vi "Login-Window-Core.vi"(5 "Cluster":T1, 7 "PwdMgr":refnum<class "PwdMgr.lvclass">, 8 "Error in":errorcluster caption="Error in (no error)", 9 "Fit to Large Dec?(T)":bool=TRUE, 11 "Options":T2={"HideMain(T)"=TRUE, "RetryAllowed(T)"=TRUE, "LastUserToINI(T)"=TRUE, "Titlebar(T)"=TRUE}) -> (0 "Error out":errorcluster={"status"=TRUE, "code"=43, "source"="Operation cancelled by user."}, 1 "Valid User":bool, 3 "User Info":T3={"UserName"="", "Password"="", "Role"=enum."Admin"})   [LabVIEW 2020, in "Login-UI.lvlib"]
uses:
  Login-UI.lvlib
  _Typedef/User-Info.ctl
  _Typedef/User-Role.ctl
  Login-Options.ctl
  PwdMgr/PwdMgr.lvclass
  <vilib>/event_ctls.llb/eventvkey.ctl
  82dbac5f-f66d-497b-81a9-0f95a8baf484.vi
  <resource>/dialog/lvconfig.llb/LV Config Write String.vi
  <resource>/dialog/lvconfig.llb/LV Config Read String.vi
  <userlib>/NEVSTOP-Programming-Palette/_openG/_reuse_openG_nevstop.lvlib
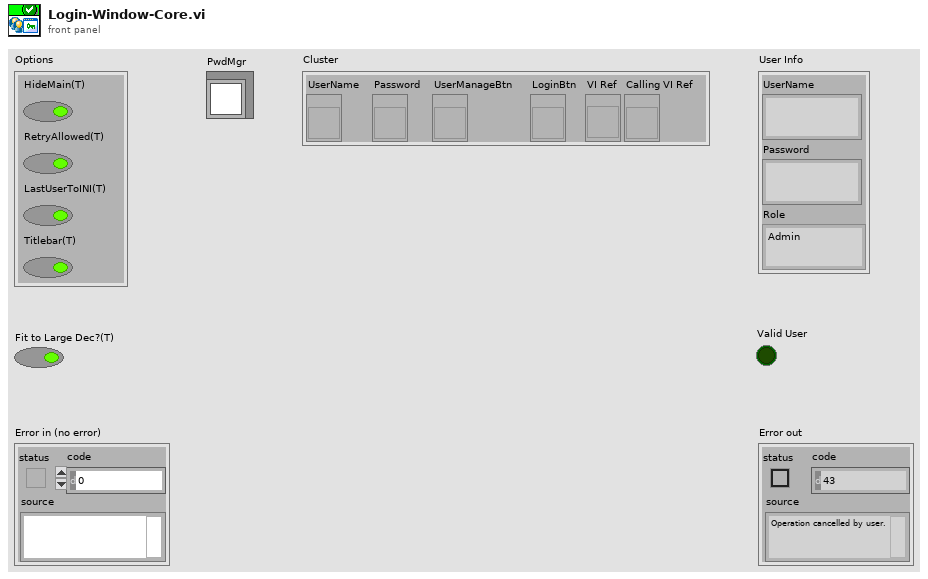
[diagram p1: front panel]
types:
  T1 = cluster{"UserName":refnum<vi>, "Password":refnum<vi>, "UserManageBtn":refnum<vi>, "LoginBtn":refnum<vi>, "VI Ref":refnum<vi>, "Calling VI Ref":refnum<vi>}
  T2 = typedef "Login-UI.lvlib/Login-Options.ctl" = cluster{"HideMain(T)":bool, "RetryAllowed(T)":bool, "LastUserToINI(T)":bool, "Titlebar(T)":bool}
  T3 = typedef "Login-UI.lvlib/User-Info.ctl" = cluster{"UserName":string, "Password":string, "Role":T4}
  T4 = typedef "Login-UI.lvlib/User-Role.ctl" = enum16{"INVALID", "Operator", "Engineer", "Admin", "Anonymous"}
  T5 = typedef "eventvkey.ctl" = enum16{"ASCII", "Enter", "Return", "Shift", "Ctrl", "Alt", "Cmd", "Opt", "Caps", "NumLock", "Clear", "Break", "Up", "Down", "Left", "Right", "Insert", "Delete", "Home", "End", "PageUp", "PageDown", "Escape", "Help", "Pause", "ScrollLock", "F1", "F2", "F3", "F4", "F5", "F6", "F7", "F8", "F9", "F10", "F11", "F12", "F13", "F14", "F15", "F16", "F17", "F18", "F19", "F20", "F21", "F22", "F23", "F24", "Play", "VolumeUp", "VolumeDown", "Mute", "Two Byte Char"}
  T6 = enum32{"Invalid", "Standard", "Closed", "Hidden", "Minimized", "Maximized"}
  T7 = enum32{"invalid app kind", "Development System", "Run Time System", "Student Edition", "Embedded LabVIEW", "Evaluation", "Custom"}
  T8 = cluster{"Core":cluster{"Current VI Reference":refnum<vi>, "Close Panel on Exit?":bool}, "Options":T2, "Calling VI's Ref":refnum<vi>, "Calling VI's FP.State":enum32{"Invalid", "Standard", "Closed", "Hidden", "Minimized", "Maximized"}, "Result":cluster{"LoginSuccess":bool, "error":errorcluster, "User Info":T3}, "UserName":string, "Password":string, "StringRefs":refnum<vi>[]}
  T9 = cluster{"LoginSuccess":bool, "error":errorcluster, "User Info":T3}
  T10 = cluster{"Current VI Reference":refnum<vi>, "Close Panel on Exit?":bool}
  T11 = cluster{bool, "code":i32, "String to Prepend to source (\"\")":string}
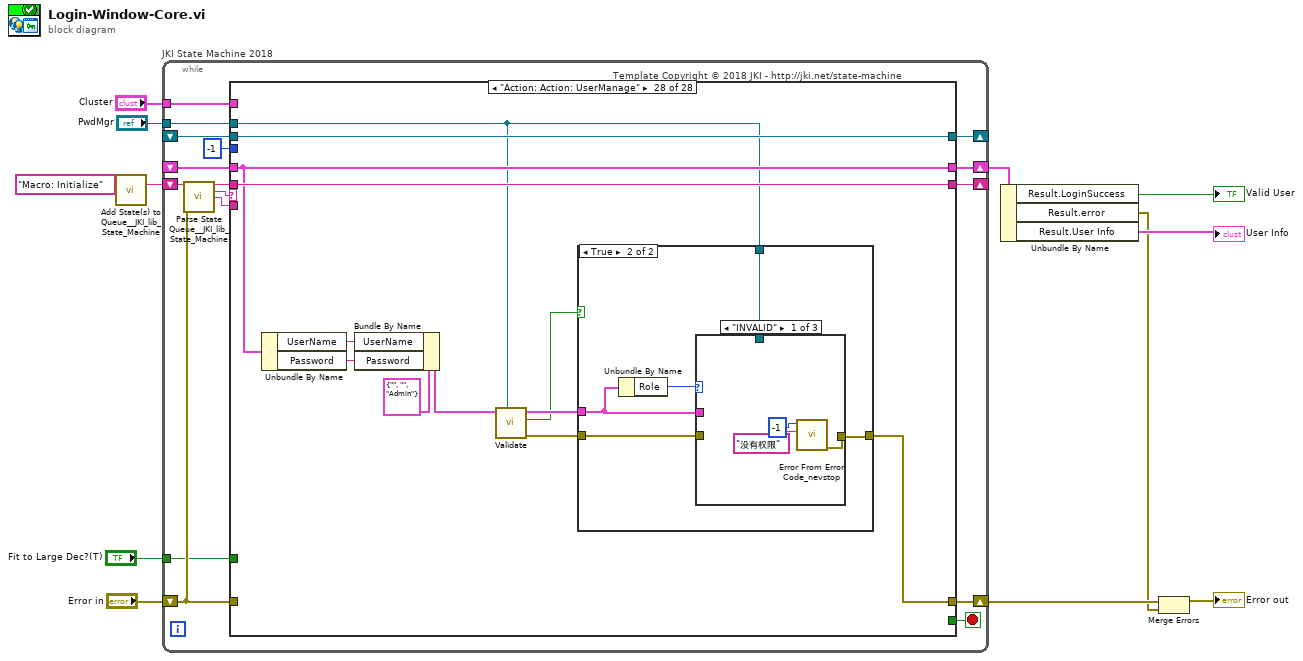
[diagram p0: block diagram]
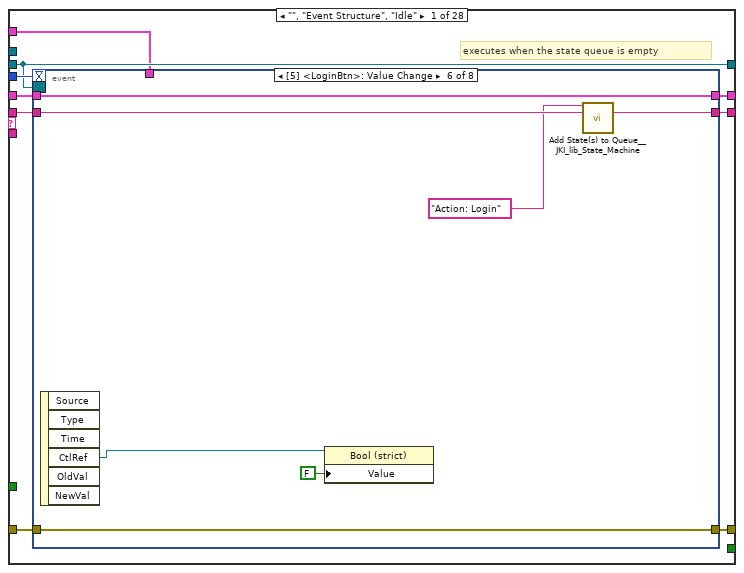
[diagram p2: hidden frame]
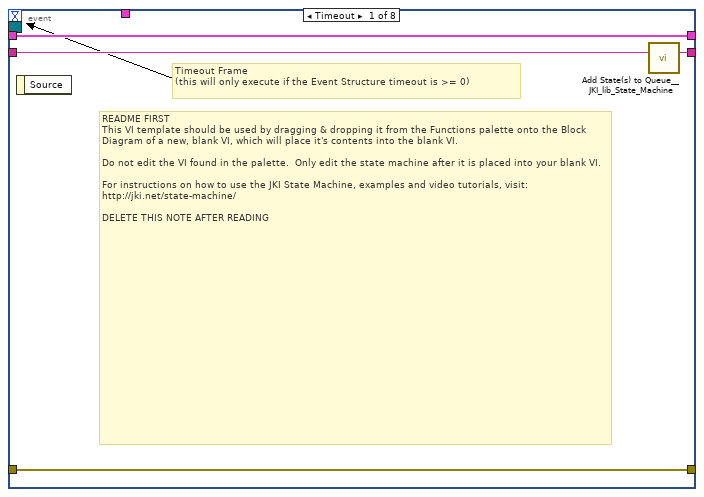
[diagram p3: hidden frame]
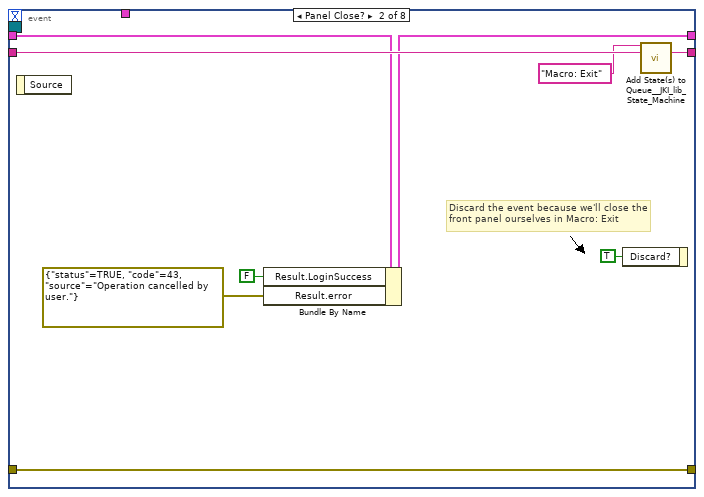
[diagram p4: hidden frame]
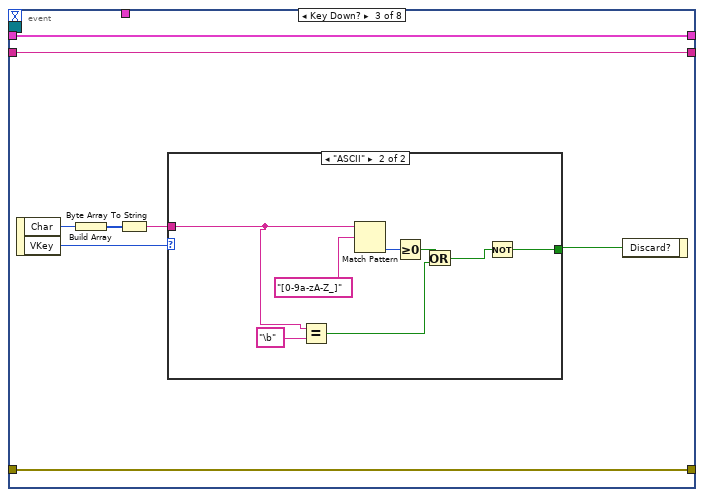
[diagram p5: hidden frame]
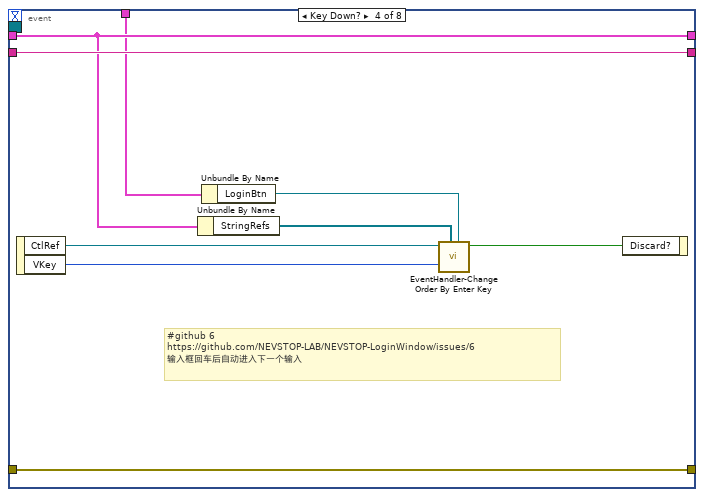
[diagram p7: hidden frame]
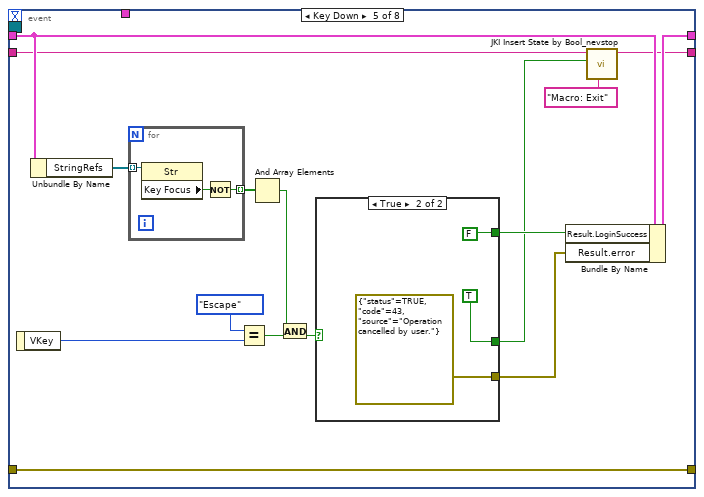
[diagram p8: hidden frame]
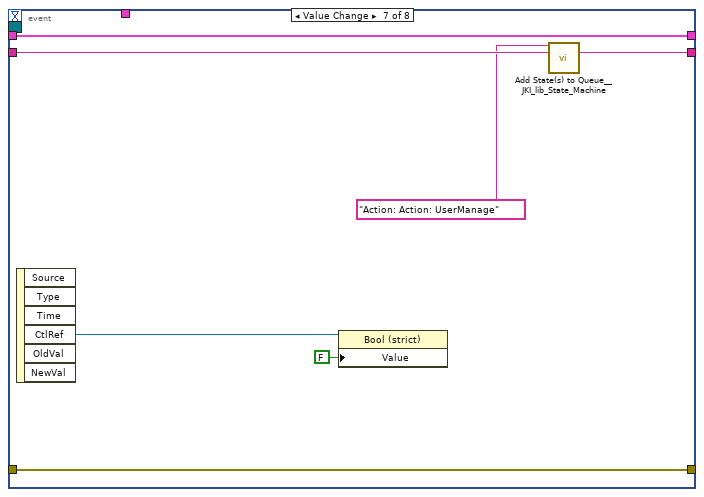
[diagram p10: hidden frame]
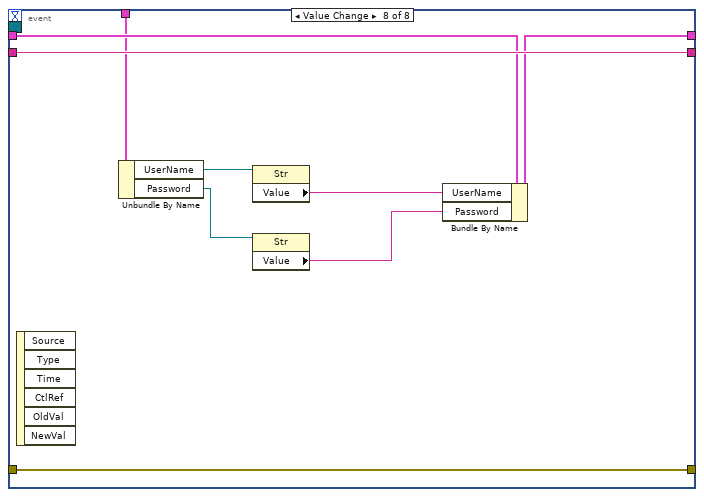
[diagram p11: hidden frame]
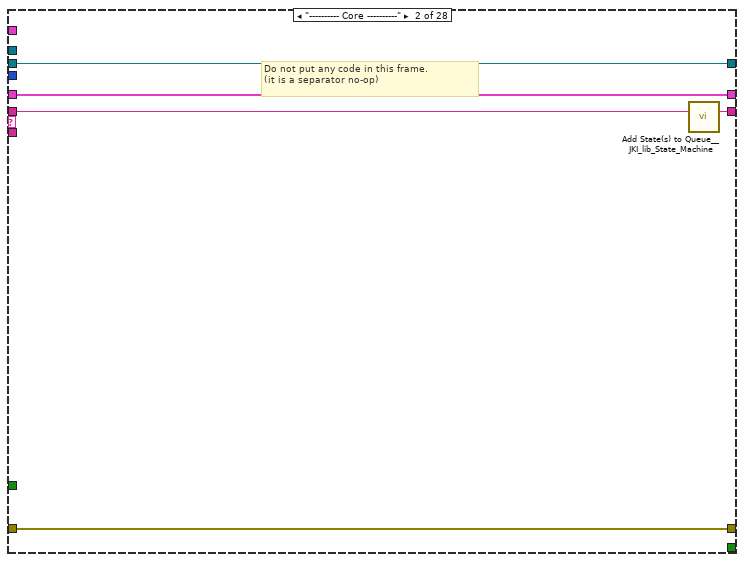
[diagram p12: hidden frame]
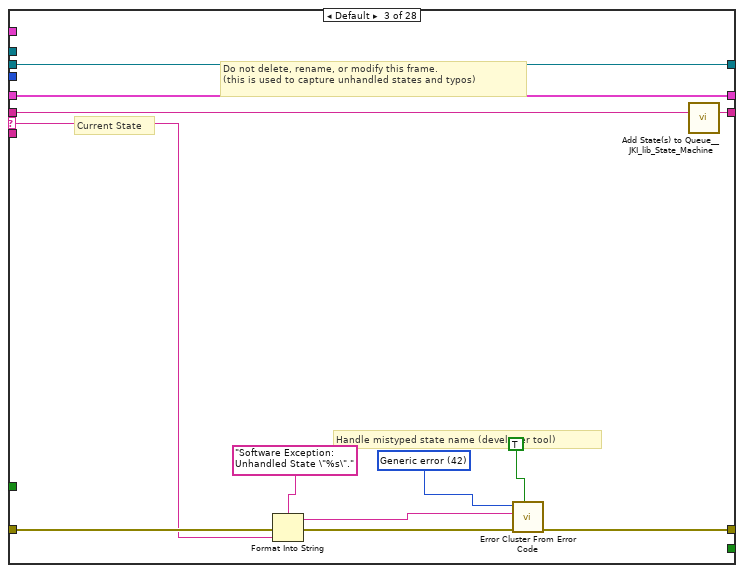
[diagram p13: hidden frame]
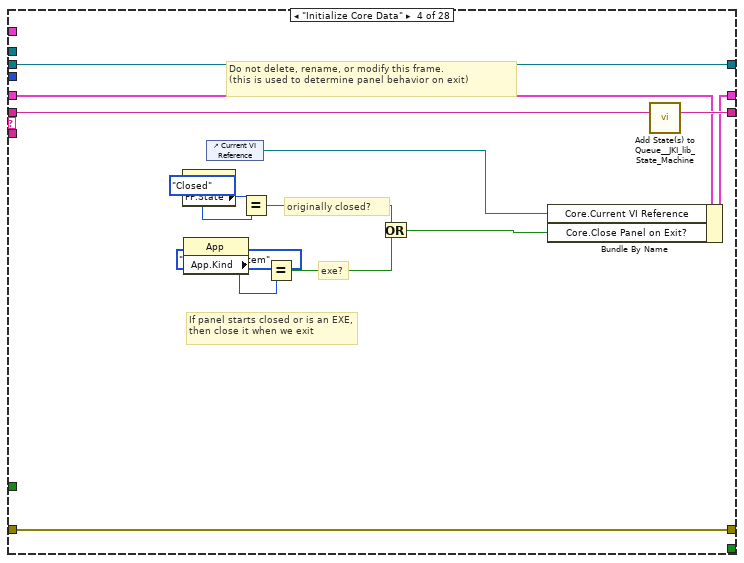
[diagram p14: hidden frame]
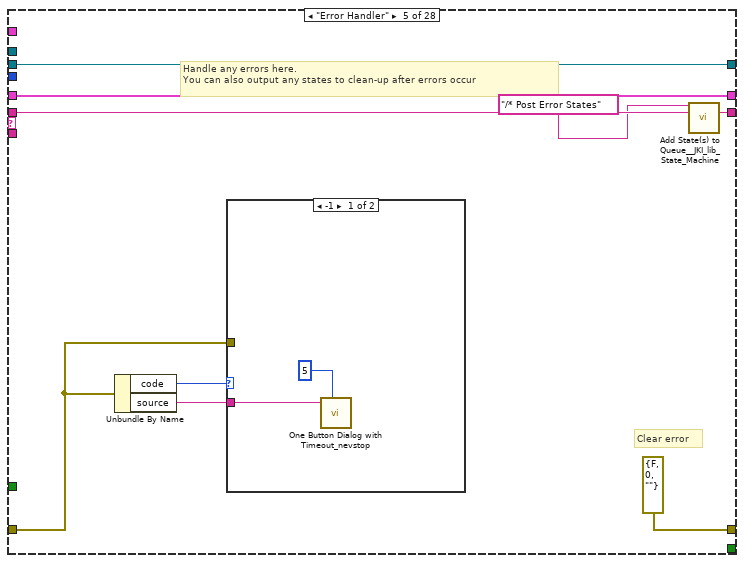
[diagram p15: hidden frame]
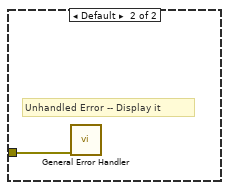
[diagram p16: hidden frame]
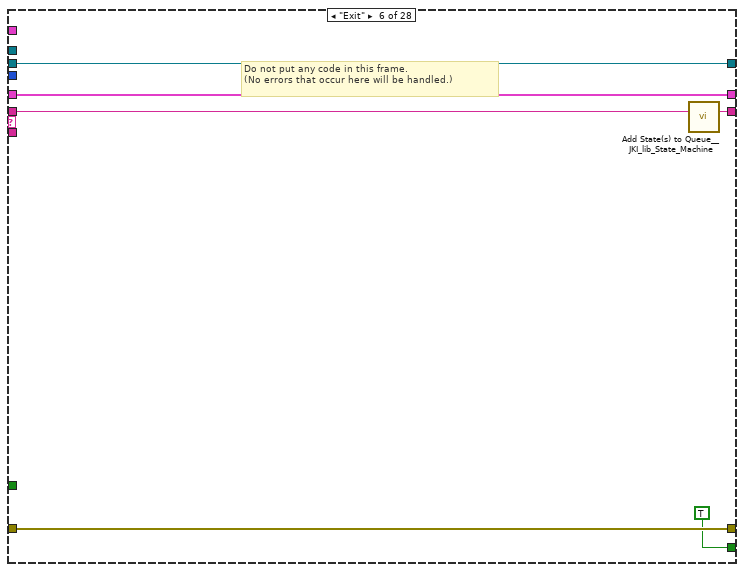
[diagram p17: hidden frame]
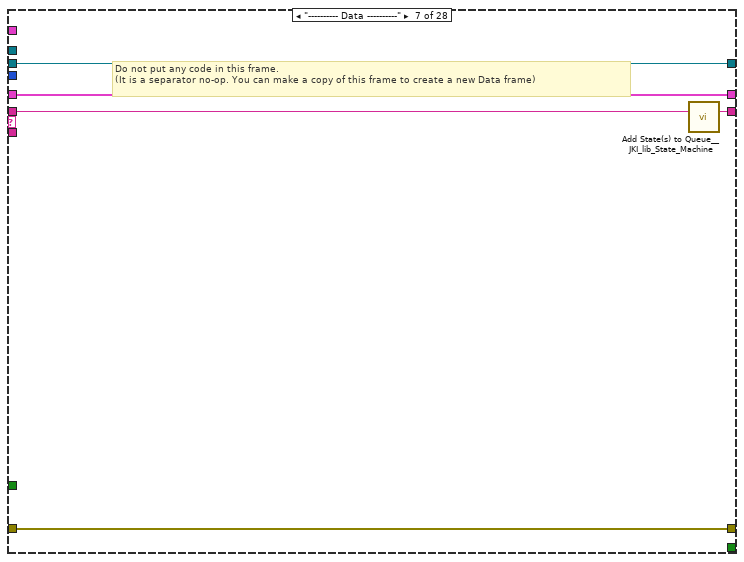
[diagram p18: hidden frame]
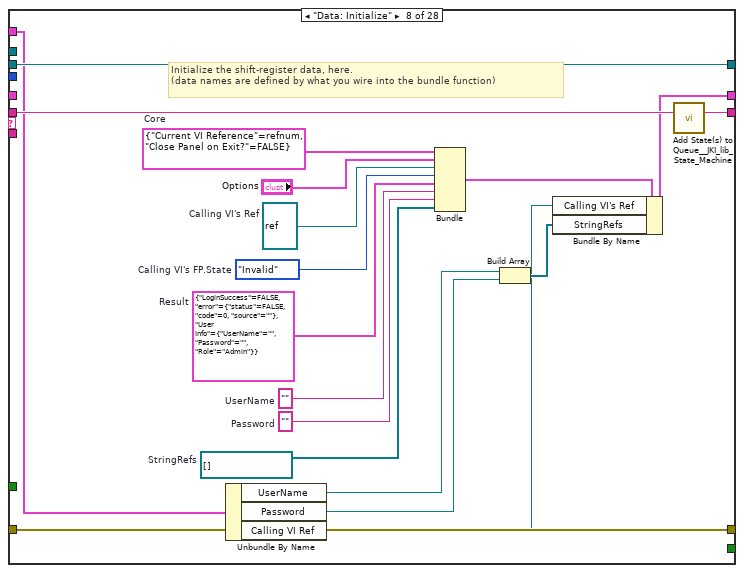
[diagram p19: hidden frame]
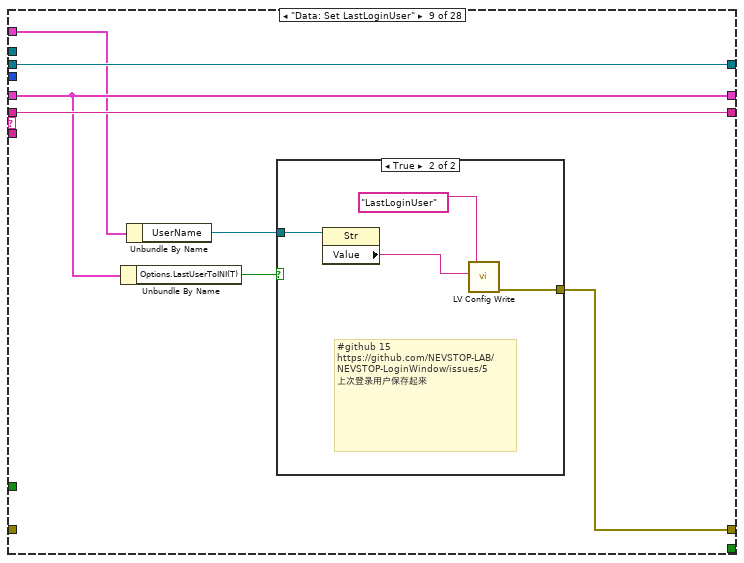
[diagram p20: hidden frame]
diagram:
  n1 = call <vilib>:"Add State(s) to Queue__JKI_lib_State_Machine.vi"("State(s) in (\"\")"="Macro: Initialize") -> ("States Out"=w10:string)  [unwired: 14 in]
  n2 = while "JKI State Machine 2018" {
    shift-right: [w21] -> w7
    shift-left: _ -> [w20]
    shift-right: [w24] -> w8
    shift-left: "Error in" -> [w18]
    shift-right: [w23] -> _
    shift-left: w10 -> [w25]
    shift-right: [w17] -> _
    shift-left: _ -> [w16]
    tunnel: "PwdMgr" -> [w15]
    tunnel: "Cluster" -> [w14]
    tunnel: "Fit to Large Dec?(T)" -> [w13]
    stop <- w22 stop-if-true
    # "Template Copyright © 2018 JKI - http://jki.net/state-machine"
    n3 = call <vilib>:"Parse State Queue__JKI_lib_State_Machine.vi"("State Queue"=w25, "Error In (no error)"=w18) -> ("Remaining States"=w27:string, "Current State"=w28:string, "Arguments"=w26:string)  [unwired: 11 in]
    n4 = case shown="\"Action: Action: UserManage\"" w28 {
      selector: w28 -> [_ _ w127 _ _ _ _ _ _ _ _ _ _ _ _ _ _ _ _ _ _ _ _ _ _ _ _ _]
      tunnel: w27 -> [w37 w125 w131 w151 w160 w169 w174 w193 w200 w211 w216 w230 w236 w241 w251 w261 w273 w347 w359 w373 w386 w392 w398 w409 w414 w433 w447 w459]
      tunnel: w26 -> [_ _ _ _ _ _ _ _ _ _ _ _ _ _ _ w256 w267 _ _ _ _ _ _ _ _ _ _ _]
      tunnel: w20 -> [w35 w122 w129 w144 w157 w167 w171 _ w198 w206 w213 w219 w234 w238 w249 w259 w269 w345 w356 w371 w384 w389 w395 w406 w411 w425 w443 w456]
      tunnel: [w34 w123 w133 w148 errorcluster {"status"=FALSE, "code"=0, "source"=""} ("error out") w166 w172 w190 w196 w207 w214 w227 w231 w239 w246 w257 w270 w343 w360 w374 w387 w390 w396 w407 w412 w431 w445 w452] -> w24
      tunnel: w18 -> [w33 w123 w132 w148 w154 w166 w172 w190 _ w208 w214 _ w232 w239 _ w258 w271 _ w360 w374 w387 w390 w396 w407 w412 w431 w445 _]
      tunnel: [w36 w124 w130 w150 w159 w168 w173 w192 w200 w210 w215 w229 w235 w240 w250 w260 w272 w347 w359 w373 w386 w391 w397 w408 w413 w432 w446 w459] -> w23
      tunnel: [_ _ _ _ _ TRUE _ _ _ _ _ _ _ _ _ _ _ _ _ _ _ _ _ _ _ _ _ _] -> w22
      tunnel: [w32 w122 w129 w149 w157 w167 w171 w184 w198 w206 w213 w219 w234 w238 w249 w259 w269 w345 w354 w371 w384 w389 w395 w406 w411 w421 w441 w456] -> w21
      tunnel: -1 ("Timeout") -> [w31 _ _ _ _ _ _ _ _ _ _ _ _ _ _ _ _ _ _ _ _ _ _ _ _ _ _ _]
      tunnel: [w30 w121 w126 w138 w155 w164 w170 w188 w199 w205 w212 w228 w233 w237 w248 w255 w266 w346 w358 w372 w385 w388 w393 w399 w410 w430 w444 w458] -> w17
      tunnel: w16 -> [w30 w121 w126 w138 w155 w164 w170 w188 w199 w205 w212 _ w233 w237 w248 w255 w266 w346 w358 w372 w385 w388 w393 w399 w410 w430 w444 w458]
      tunnel: w15 -> [_ _ _ _ _ _ _ _ _ _ _ _ _ _ _ _ _ _ _ _ _ _ _ _ _ w418 _ w448]
      tunnel: w14 -> [w29 _ _ _ _ _ _ w178 w195 _ _ w226 _ _ w244 _ _ w342 _ _ _ _ _ _ _ _ _ _]
      tunnel: w13 -> [_ _ _ _ _ _ _ _ _ _ _ _ _ _ w242 _ _ _ _ _ _ _ _ _ _ _ _ _]
      frame "", "Event Structure", "Idle" {
        # "executes when the state queue is empty"
        n5 = event shown="[5] <LoginBtn>: Value Change" {
          selector: w30 -> [_ _ _ _ _ _ _ _]
          dyn-events: _ -> [_ _ _ _ _ _ _ _]
          timeout: w31 -> [_ _ _ _ _ _ _ _]
          tunnel: w37 -> [w41 w50 w58 w75 w78 w101 w108 w120]
          tunnel: [w40 w49 w58 w75 w79 w102 w109 w120] -> w36
          tunnel: w35 -> [w38 w47 w56 w70 w84 w103 w110 w118]
          tunnel: [w39 w48 w57 w74 w91 w104 w111 w119] -> w34
          tunnel: w33 -> [w39 w48 w57 w74 w91 w104 w111 w119]
          tunnel: [w38 w44 w56 w70 w82 w103 w110 w117] -> w32
          tunnel: w29 -> [_ _ _ w68 _ _ _ w116]
          event Timeout {
            # "README FIRST\nThis VI template should be used by dragging & dropping it from the Functions palette onto the Block Diagram of a new, blank VI, which will place it's contents into the blank VI.\n\nDo not edit the VI found in the palette.  Only edit the state machine after it is placed into your blank VI.\n\nFor instructions on how to use the JKI State Machine, examples and video tutorials, visit:\nhttp://jki.net/state-machine/\n\nDELETE THIS NOTE AFTER READING"
            # "Timeout Frame\n(this will only execute if the Event Structure timeout is >= 0)"
            n6 = event-data() -> ()  [unwired: 1 in, 1 out]
            n7 = call <vilib>:"Add State(s) to Queue__JKI_lib_State_Machine.vi"("State(s) in (\"\")"=w41) -> ("States Out"=w40:string)  [unwired: 14 in]
          }
          event Panel Close? {
            # "Discard the event because we'll close the front panel ourselves in Macro: Exit"
            n8 = event-data() -> ()  [unwired: 1 in, 1 out]
            n9 = Bundle By Name(cluster=w47, "Result.LoginSuccess"=FALSE, "Result.error"=errorcluster {"status"=TRUE, "code"=43, "source"="Operation cancelled by user."} ("error in")) -> (w44:T8)
            n10 = event-data("Discard?"=TRUE) -> ()  [unwired: 1 in, 1 out]
            n11 = call <vilib>:"Add State(s) to Queue__JKI_lib_State_Machine.vi"("State(s) in Front (\"\")"="Macro: Exit", "State(s) in (\"\")"=w50) -> ("States Out"=w49:string)  [unwired: 13 in]
          }
          event Key Down? {
            n12 = event-data() -> ("Char"=w53:i16, "VKey"=w52:T5)  [unwired: 1 in]
            n13 = Build Array(w53) -> (w54:i16[])
            n14 = Byte Array To String(unsigned byte array=w54) -> (string=w55:string)
            n15 = case shown="\"ASCII\"" w52 {
              tunnel: [_ w59] -> w51
              tunnel: w55 -> [_ w62]
              frame Default {
              }
              frame "ASCII" {
                n16 = Equal?(x=w62, y="\b" ("regular expression")) -> (x = y?=w60:bool)
                n17 = Match Pattern(string=w62, regular expression="[0-9a-zA-Z_]") -> (offset past match=w65:i32)  [unwired: 1 in, 3 out]
                n18 = Greater Or Equal To 0?(x=w65) -> (x >= 0?=w64:bool)
                n19 = Or(x=w64, y=w60) -> (x .or. y?=w61:bool)
                n20 = Not(x=w61) -> (.not. x?=w59:bool)
              }
            }
            n21 = event-data("Discard?"=w51) -> ()  [unwired: 1 in, 1 out]
          }
          event Key Down? {
            # "#github 6\nhttps://github.com/NEVSTOP-LAB/NEVSTOP-LoginWindow/issues/6\n输入框回车后自动进入下一个输入"
            n22 = event-data() -> ("CtlRef"=w72:refnum<vi>, "VKey"=w73:T5)  [unwired: 1 in]
            n23 = Unbundle By Name(w70) -> ("StringRefs"=w69:refnum<vi>[])
            n24 = Unbundle By Name(w68) -> ("LoginBtn"=w67:refnum<vi>)
            n25 = call "EventHandler-Change Order By Enter Key.vi"("Next Ctrl"=w67, "Controls for changing order"=w69, "VKey"=w73, "Event Control"=w72) -> ("Discard?"=w71:bool)  [unwired: 7 in]
            n26 = event-data("Discard?"=w71) -> ()  [unwired: 1 in, 1 out]
          }
          event Key Down {
            n27 = event-data() -> ("VKey"=w85:T5)  [unwired: 1 in]
            n28 = Unbundle By Name(w84) -> ("StringRefs"=w83:refnum<vi>[])
            n29 = for {
              tunnel: w83 -> [w94] mode=indexing
              tunnel: [w92] -> w89 mode=indexing
              n30 = property class="Str"(reference=w94) -> ("Key Focus"=w93:bool)  [unwired: 1 in, 2 out]
              n31 = Not(x=w93) -> (.not. x?=w92:bool)
            }
            n32 = Equal?(x=eventvkey."Escape", y=w85) -> (x = y?=w87:bool)
            n33 = And Array Elements(Boolean array=w89) -> (logical AND=w90:bool)
            n34 = And(x=w90, y=w87) -> (x .and. y?=w88:bool)
            n35 = case shown="True" w88 {
              tunnel: [_ TRUE ("Discard?")] -> w77
              tunnel: [_ FALSE ("Discard?")] -> w81
              tunnel: [_ errorcluster {"status"=TRUE, "code"=43, "source"="Operation cancelled by user."} ("error in")] -> w80
              frame False {
              }
              frame True {
              }
            }
            n36 = Bundle By Name(cluster=w84, "Result.LoginSuccess"=w81, "Result.error"=w80) -> (w82:T8)
            n37 = call <userlib>:"JKI Insert State by Bool_nevstop.vi"("TRUE(Empty)"="Macro: Exit", "Bool"=w77, "Remaining States"=w78) -> ("States Out"=w79:string)  [unwired: 8 in]
          }
          event Value Change {
            n38 = event-data() -> ("CtlRef"=w99:refnum<vi>)  [unwired: 1 in, 5 out]
            n39 = property class="Bool (strict)"(reference=w99, "Value"=FALSE) -> ()  [unwired: 1 in, 2 out]
            n40 = call <vilib>:"Add State(s) to Queue__JKI_lib_State_Machine.vi"("State(s) in Front (\"\")"="Action: Login" ("State(s) in Front (\"\")"), "State(s) in (\"\")"=w101) -> ("States Out"=w102:string)  [unwired: 13 in]
          }
          event Value Change {
            n41 = event-data() -> ("CtlRef"=w106:refnum<vi>)  [unwired: 1 in, 5 out]
            n42 = property class="Bool (strict)"(reference=w106, "Value"=FALSE) -> ()  [unwired: 1 in, 2 out]
            n43 = call <vilib>:"Add State(s) to Queue__JKI_lib_State_Machine.vi"("State(s) in Front (\"\")"="Action: Action: UserManage" ("State(s) in Front (\"\")"), "State(s) in (\"\")"=w108) -> ("States Out"=w109:string)  [unwired: 13 in]
          }
          event Value Change {
            n44 = event-data() -> ()  [unwired: 1 in, 6 out]
            n45 = Unbundle By Name(w116) -> ("UserName"=w115:refnum<vi>, "Password"=w114:refnum<vi>)
            n46 = property class="Str"(reference=w115) -> ("Value"=w112:string)  [unwired: 1 in, 2 out]
            n47 = property class="Str"(reference=w114) -> ("Value"=w113:string)  [unwired: 1 in, 2 out]
            n48 = Bundle By Name(cluster=w118, "UserName"=w112, "Password"=w113) -> (w117:T8)
          }
        }
      }
      frame "---------- Core ----------" {
        # "Do not put any code in this frame.\n(it is a separator no-op)"
        n49 = call <vilib>:"Add State(s) to Queue__JKI_lib_State_Machine.vi"("State(s) in (\"\")"=w125) -> ("States Out"=w124:string)  [unwired: 14 in]
      }
      frame Default {
        w136 = 42 items=["No error", "Argument error", "Memory is full", "Out of zone", "End of file", "File already open", "Generic file I/O error", "File not found", "File permission error", "Disk is full", "Duplicate path", "Too many files open", "System feature not enabled", "Resource file not found", "Cannot add resource", "Resource not found", "Image not found", "Image memory error", "Pen does not exist", "Config type invalid", "Config token not found", "Config parse error", "Config memory error", "Bad external code format", "Bad external code offset", "External code not present", "Null window", "Destroy window error", "Null menu", "Print aborted", "Bad print record", "Print driver error", "Windows error during printing", "Memory error during printing", "Print dialog error", "Generic print error", "Invalid device refnum", "Device not found", "Device parameter error", "Device unit error", "Cannot open device", "Device call aborted", "Generic error", "Cancelled by user", "Object ID too low", "Object ID too high", "Object not in heap", "Unknown heap", "Unknown object (invalid DefProc)", "Unknown object (DefProc not in table)", "Message out of range", "Invalid (null) method", "Unknown message", "Manager call not supported", "Bad address", "Network operation in progress", "Network operation timed out", "Connection is busy", "Network attribute not supported", "Network error", "Address in use", "System out of memory", "Connection aborted", "Connection refused", "Not connected", "Already connected", "Connection closed", "Initialization error (interapplication manager)", "Bad occurrence", "Wait on unbound occurrence handler", "Occurrence queue overflow", "Datalog type conflict", "Unused", "Unrecognized type (interapplication manager)", "Memory corrupt", "Failed to make temporary DLL", "Old CIN version", "Drag socket not found", "Failed to load drop-object", "Failed to register OLE object", "Failed to release OLE object", "Format specifier type mismatch", "Unknown format specifier", "Too few format specifiers", "Too many format specifiers", "Scan failed", "Newer CIN version", "Error converting to variant", "Runtime menu error", "Password tampered", "Variant attribute not found", "Incompatible variant data type", "Event data is not available", "Event Store is not present", "Occurrence is not found", "Event Queue is not created", "Event info is not available", "Refnum passed is NULL", "Error retrieving Class GUID", "Error retrieving CoClass GUID", "Error retrieving TypeLib GUID.", "Bad built application magic bytes.", "Specific driver is different from the specific driver associated with the Logical Name.", "There is no session opened to the class driver.", "Max Error", "MAX - Error with config objects", "MAX - Error loading configuration", "MAX - Group not supported"]
        # "Current State"
        # "Do not delete, rename, or modify this frame.\n(this is used to capture unhandled states and typos)"
        # "Handle mistyped state name (developer tool)"
        n50 = Format Into String(format string="Software Exception: Unhandled State \"%s\"." ("message"), error in=w132, w127) -> (resulting string=w135:string, error out=w134:errorcluster)  [unwired: 1 in]
        n51 = call <vilib>:"Error Cluster From Error Code.vi"("show call chain? (False)"=TRUE, "error in (no error)"=w134, "error message (\"\")"=w135, "error code (0)"=w136) -> ("error out"=w133:errorcluster)  [unwired: 5 in]
        n52 = call <vilib>:"Add State(s) to Queue__JKI_lib_State_Machine.vi"("State(s) in (\"\")"=w131) -> ("States Out"=w130:string)  [unwired: 14 in]
      }
      frame "Initialize Core Data" {
        # "Do not delete, rename, or modify this frame.\n(this is used to determine panel behavior on exit)"
        # "originally closed?"
        # "exe?"
        # "If panel starts closed or is an EXE, then close it when we exit"
        n53 = property class="VI"() -> ("FP.State"=w141:T6)  [unwired: 2 in, 2 out]
        n54 = property class="App"() -> ("App.Kind"=w147:T7)  [unwired: 2 in, 2 out]
        n55 = control-ref of="Current VI Reference"() -> (w142:refnum<vi>)
        n56 = Equal?(x=w141, y=T6."Closed" ("Front Panel Window:State")) -> (x = y?=w139:bool)
        n57 = Equal?(x=w147, y=T7."Run Time System" ("Application:Kind")) -> (x = y?=w145:bool)
        n58 = Or(x=w139, y=w145) -> (x .or. y?=w143:bool)
        n59 = Bundle By Name(cluster=w144, "Core.Current VI Reference"=w142, "Core.Close Panel on Exit?"=w143) -> (w149:T8)
        n60 = call <vilib>:"Add State(s) to Queue__JKI_lib_State_Machine.vi"("State(s) in (\"\")"=w151) -> ("States Out"=w150:string)  [unwired: 14 in]
      }
      frame "Error Handler" {
        # "Handle any errors here.\nYou can also output any states to clean-up after errors occur"
        # "Clear error"
        n61 = Unbundle By Name(w154) -> ("code"=w153:i32, "source"=w152:string)
        n62 = case shown="-1" w153 {
          tunnel: w154 -> [_ w163]
          tunnel: w152 -> [w162 _]
          frame -1 {
            n63 = call <userlib>:"One Button Dialog with Timeout_nevstop.vi"("message"=w162, "Btn Timeout(-1 s)"=5) -> ()  [unwired: 7 in, 1 out]
          }
          frame Default {
            # "Unhandled Error -- Display it"
            n64 = call <vilib>:"General Error Handler.vi"("error in (no error)"=w163) -> ()  [unwired: 10 in, 5 out]
          }
        }
        n65 = call <vilib>:"Add State(s) to Queue__JKI_lib_State_Machine.vi"("State(s) in Front (\"\")"="/* Post Error States", "State(s) in (\"\")"=w160) -> ("States Out"=w159:string)  [unwired: 13 in]
      }
      frame "Exit" {
        # "Do not put any code in this frame.\n(No errors that occur here will be handled.)"
        n66 = call <vilib>:"Add State(s) to Queue__JKI_lib_State_Machine.vi"("State(s) in (\"\")"=w169) -> ("States Out"=w168:string)  [unwired: 14 in]
      }
      frame "---------- Data ----------" {
        # "Do not put any code in this frame.\n(It is a separator no-op. You can make a copy of this frame to create a new Data frame)"
        n67 = call <vilib>:"Add State(s) to Queue__JKI_lib_State_Machine.vi"("State(s) in (\"\")"=w174) -> ("States Out"=w173:string)  [unwired: 14 in]
      }
      frame "Data: Initialize" {
        w180 = refnum<vi>[] []  # StringRefs
        w181 = ""  # Password
        w182 = ""  # UserName
        w183 = T9 {"LoginSuccess"=FALSE, "error"={"status"=FALSE, "code"=0, "source"=""}, "User Info"={"UserName"="", "Password"="", "Role"=enum."Admin"}}  # Result
        w185 = T6."Invalid"  # Calling VI's FP.State
        w186 = refnum<vi> refnum  # Calling VI's Ref
        w189 = T10 {"Current VI Reference"=refnum, "Close Panel on Exit?"=FALSE}  # Core
        # "Initialize the shift-register data, here.\n(data names are defined by what you wire into the bundle function)"
        n68 = Unbundle By Name(w178) -> ("UserName"=w177:refnum<vi>, "Password"=w176:refnum<vi>, "Calling VI Ref"=w175:refnum<vi>)
        n69 = Bundle("Core"=w189, "Options"="Options", "Calling VI's Ref"=w186, "Calling VI's FP.State"=w185, "Result"=w183, "UserName"=w182, "Password"=w181, "StringRefs"=w180) -> (w191:T8)  [unwired: 1 in]
        n70 = Build Array(w177, w176) -> (w179:refnum<vi>[])
        n71 = Bundle By Name(cluster=w191, "Calling VI's Ref"=w175, "StringRefs"=w179) -> (w184:T8)
        n72 = call <vilib>:"Add State(s) to Queue__JKI_lib_State_Machine.vi"("State(s) in (\"\")"=w193) -> ("States Out"=w192:string)  [unwired: 14 in]
      }
      frame "Data: Set LastLoginUser" {
        n73 = Unbundle By Name(w198) -> ("Options.LastUserToINI(T)"=w197:bool)
        n74 = Unbundle By Name(w195) -> ("UserName"=w194:refnum<vi>)
        n75 = case shown="True" w197 {
          tunnel: [_ w203] -> w196
          tunnel: w194 -> [_ w202]
          frame False {
          }
          frame True {
            # "#github 15\nhttps://github.com/NEVSTOP-LAB/NEVSTOP-LoginWindow/issues/5\n上次登录用户保存起来"
            n76 = property class="Str"(reference=w202) -> ("Value"=w201:string)  [unwired: 1 in, 2 out]
            n77 = call-poly <resource>:"LV Config Write.vi"("value"=w201, "key"="LastLoginUser") -> ("error out"=w203:errorcluster)  [unwired: 5 in]
          }
        }
      }
      frame "Data: Cleanup" {
        # "Cleanup any data and references, here.\n(this is called automatically, by the Macro: Exit)"
        n78 = Unbundle By Name(w206) -> ("Core.Current VI Reference"=w209:refnum<vi>)
        n79 = Close Reference(reference=w209, error in (no error)=w208) -> (error out=w207:errorcluster)
        n80 = call <vilib>:"Add State(s) to Queue__JKI_lib_State_Machine.vi"("State(s) in (\"\")"=w211) -> ("States Out"=w210:string)  [unwired: 14 in]
      }
      frame "---------- Events ----------" {
        # "Do not put any code in this frame.\n(It is a separator no-op. You can make a copy of this frame to create a new UI frame)"
        n81 = call <vilib>:"Add State(s) to Queue__JKI_lib_State_Machine.vi"("State(s) in (\"\")"=w216) -> ("States Out"=w215:string)  [unwired: 14 in]
      }
      frame "Events: Register" {
        n82 = Unbundle By Name(w226) -> ("UserName"=w221:refnum<vi>, "Password"=w220:refnum<vi>, "UserManageBtn"=w225:refnum<vi>, "LoginBtn"=w224:refnum<vi>, "UserName"=w223:refnum<vi>, "Password"=w222:refnum<vi>, "VI Ref"=w217:refnum<vi>)
        n83 = Unbundle By Name(w219) -> ("StringRefs"=w218:refnum<vi>[])
        n84 = register-events(w218, w221, w220, w225, w224, w223, w222, w217, w217) -> (reference out=w228:refnum<event-registration>, error out=w227:errorcluster)  [unwired: 2 in]
        n85 = call <vilib>:"Add State(s) to Queue__JKI_lib_State_Machine.vi"("State(s) in (\"\")"=w230) -> ("States Out"=w229:string)  [unwired: 14 in]
      }
      frame "Events: Unregister" {
        # "Do not put any code in this frame.\n(It is a separator no-op. You can make a copy of this frame to create a new UI frame)"
        n86 = Unregister For Events(event registration refnum=w233, error in=w232) -> (error out=w231:errorcluster)
        n87 = call <vilib>:"Add State(s) to Queue__JKI_lib_State_Machine.vi"("State(s) in (\"\")"=w236) -> ("States Out"=w235:string)  [unwired: 14 in]
      }
      frame "---------- UI ----------" {
        # "Do not put any code in this frame.\n(It is a separator no-op. You can make a copy of this frame to create a new UI frame)"
        n88 = call <vilib>:"Add State(s) to Queue__JKI_lib_State_Machine.vi"("State(s) in (\"\")"=w241) -> ("States Out"=w240:string)  [unwired: 14 in]
      }
      frame "UI: Initialize" {
        # "Initialize the User Interface, here.\n(this is called automatically, by the Macro: Init)"
        n89 = Unbundle By Name(w244) -> ("VI Ref"=w243:refnum<vi>)
        n90 = case shown="True" w242 {
          tunnel: [_ w254] -> w247
          tunnel: w243 -> [_ w252]
          frame False {
          }
          frame True {
            n91 = call <userlib>:"Fit VI window to Largest Dec_nevstop.vi"("border spacing (2 px)"=-2, "VI Ref (calling VI)"=w252) -> ("error out"=w254:errorcluster)  [unwired: 4 in, 1 out]
          }
        }
        n92 = invoke class="VI" method="Default Vals.Reinit All"(error in=w247) -> (error out=w246:errorcluster)  [unwired: 2 in, 2 out]
        n93 = call <vilib>:"Add State(s) to Queue__JKI_lib_State_Machine.vi"("State(s) in Front (\"\")"="UI: Hide Caller Panel\nUI: Set Titlebar State\n\n// User + Password 在这里初始化\nUI: Set Last Login User" ("State(s) in Front (\"\")"), "State(s) in (\"\")"=w251) -> ("States Out"=w250:string)  [unwired: 13 in]
      }
      frame "UI: Cursor Set" {
        # "Argument"
        # "Set and Unset Cursor Busy.\n(Usage: \"UI: Cursor Set >> Busy|Idle\")"
        n94 = case shown="\"Idle\", Default" w256 {
          tunnel: w258 -> [w263 w265]
          tunnel: [w262 w264] -> w257
          frame "Idle", Default {
            n95 = call <vilib>:"Unset Busy.vi"("error in (no error)"=w263) -> ("error out"=w262:errorcluster)  [unwired: 10 in]
          }
          frame "Busy" {
            n96 = call <vilib>:"Set Busy.vi"("error in (no error)"=w265) -> ("error out"=w264:errorcluster)  [unwired: 9 in, 1 out]
          }
        }
        n97 = call <vilib>:"Add State(s) to Queue__JKI_lib_State_Machine.vi"("State(s) in (\"\")"=w261) -> ("States Out"=w260:string)  [unwired: 14 in]
      }
      frame "UI: Front Panel State" {
        # "Argument"
        # "Set Front Panel Open or Closed\n(Usage: \"UI: Front Panel State >> Open|Close\")"
        n98 = Unbundle By Name(w269) -> ("Core.Current VI Reference"=w268:refnum<vi>)
        n99 = case shown="\"Minimize\", \"Minimized\"" w267 {
          tunnel: w271 -> [w279 w294 w305 w318 w331]
          tunnel: [w281 w295 w307 w320 w333] -> w270
          tunnel: w268 -> [w280 w292 w306 w319 w332]
          frame "Open", "Standard", Default {
            w274 = T6."Standard" ("State")
            n100 = property class="VI"(reference=w280, error in=w279) -> (reference out=w277:refnum<vi>, error out=w278:errorcluster, "FP.State"=w276:T6)
            n101 = Not Equal?(x=w276, y=w274) -> (x != y?=w275:bool)
            n102 = case shown="True" w275 {
              tunnel: [w285 w287] -> w281
              tunnel: w278 -> [w284 w287]
              tunnel: w277 -> [w283 _]
              tunnel: w274 -> [w282 _]
              frame True {
                n103 = invoke class="VI" method="FP.Open"(reference=w283, error in=w284, "Activate"=TRUE, "State"=w282) -> (error out=w285:errorcluster)  [unwired: 1 in, 4 out]
              }
              frame False {
              }
            }
          }
          frame "Close", "Closed" {
            n104 = property class="VI"(reference=w292, error in=w294) -> (reference out=w291:refnum<vi>, error out=w293:errorcluster, "FP.State"=w289:T6)
            n105 = Not Equal?(x=w289, y=T6."Closed" ("Front Panel Window:State")) -> (x != y?=w288:bool)
            n106 = case shown="True" w288 {
              tunnel: [w296 w299] -> w295
              tunnel: w293 -> [w296 w298]
              tunnel: w291 -> [_ w297]
              frame False {
              }
              frame True {
                n107 = invoke class="VI" method="FP.Close"(reference=w297, error in=w298) -> (error out=w299:errorcluster)  [unwired: 1 in, 2 out]
              }
            }
          }
          frame "Hidden", "Hide" {
            w300 = T6."Hidden" ("State")
            n108 = property class="VI"(reference=w306, error in=w305) -> (reference out=w303:refnum<vi>, error out=w304:errorcluster, "FP.State"=w302:T6)
            n109 = Not Equal?(x=w302, y=w300) -> (x != y?=w301:bool)
            n110 = case shown="True" w301 {
              tunnel: [w311 w312] -> w307
              tunnel: w304 -> [w310 w312]
              tunnel: w303 -> [w309 _]
              tunnel: w300 -> [w308 _]
              frame True {
                n111 = invoke class="VI" method="FP.Open"(reference=w309, error in=w310, "State"=w308) -> (error out=w311:errorcluster)  [unwired: 2 in, 4 out]
              }
              frame False {
              }
            }
          }
          frame "Minimize", "Minimized" {
            w313 = T6."Minimized" ("State")
            n112 = property class="VI"(reference=w319, error in=w318) -> (reference out=w316:refnum<vi>, error out=w317:errorcluster, "FP.State"=w315:T6)
            n113 = Not Equal?(x=w315, y=w313) -> (x != y?=w314:bool)
            n114 = case shown="True" w314 {
              tunnel: [w324 w325] -> w320
              tunnel: w317 -> [w323 w325]
              tunnel: w316 -> [w322 _]
              tunnel: w313 -> [w321 _]
              frame True {
                n115 = invoke class="VI" method="FP.Open"(reference=w322, error in=w323, "State"=w321) -> (error out=w324:errorcluster)  [unwired: 2 in, 4 out]
              }
              frame False {
              }
            }
          }
          frame "Maximize", "Maximized" {
            w326 = T6."Maximized" ("State")
            n116 = property class="VI"(reference=w332, error in=w331) -> (reference out=w329:refnum<vi>, error out=w330:errorcluster, "FP.State"=w328:T6)
            n117 = Not Equal?(x=w328, y=w326) -> (x != y?=w327:bool)
            n118 = case shown="True" w327 {
              tunnel: [w337 w338] -> w333
              tunnel: w330 -> [w336 w338]
              tunnel: w329 -> [w335 _]
              tunnel: w326 -> [w334 _]
              frame True {
                n119 = invoke class="VI" method="FP.Open"(reference=w335, error in=w336, "State"=w334) -> (error out=w337:errorcluster)  [unwired: 2 in, 4 out]
              }
              frame False {
              }
            }
          }
        }
        n120 = call <vilib>:"Add State(s) to Queue__JKI_lib_State_Machine.vi"("State(s) in (\"\")"=w273) -> ("States Out"=w272:string)  [unwired: 14 in]
      }
      frame "UI: Set Last Login User" {
        # "#github 15\nhttps://github.com/NEVSTOP-LAB/NEVSTOP-LoginWindow/issues/5\n上次登录用户保存起来"
        n121 = Unbundle By Name(w345) -> ("Options.LastUserToINI(T)"=w344:bool)
        n122 = Unbundle By Name(w342) -> ("Password"=w341:refnum<vi>, "UserName"=w339:refnum<vi>)
        n123 = case shown="True" w344 {
          tunnel: [_ w350] -> w343
          tunnel: w339 -> [_ w349]
          frame False {
          }
          frame True {
            n124 = call-poly <resource>:"LV Config Read.vi"("default value"="", "key"="LastLoginUser") -> ("error out"=w350:errorcluster, "value"=w348:string)  [unwired: 3 in, 1 out]
            n125 = property class="Str"(reference=w349, "Value"=w348) -> ()  [unwired: 1 in, 2 out]
          }
        }
        n126 = property class="Str"(reference=w341, "Value"="" ("Password")) -> ()  [unwired: 1 in, 2 out]
      }
      frame "UI: Hide Caller Panel" {
        n127 = Unbundle By Name(w356) -> ("Calling VI's Ref"=w355:refnum<vi>, "Options.HideMain(T)"=w357:bool)
        n128 = flat-sequence {
          tunnel: [w363] -> w353
          tunnel: w357 -> [w362]
          tunnel: w355 -> [w361]
          frame #0 {
            n129 = case shown="True" w362 {
              tunnel: [_ w365] -> w363
              tunnel: w361 -> [_ w364]
              frame False {
              }
              frame True {
                n130 = property class="VI"(reference=w364, "FP.State"=T6."Hidden" ("Front Panel Window:State")) -> ("FP.State"=w365:T6)  [unwired: 1 in, 2 out]
              }
            }
          }
        }
        n131 = Bundle By Name(cluster=w356, "Calling VI's FP.State"=w353) -> (w354:T8)
      }
      frame "UI: Restore Caller Panel State" {
        n132 = Unbundle By Name(w371) -> ("Calling VI's Ref"=w370:refnum<vi>, "Options.HideMain(T)"=w368:bool, "Calling VI's FP.State"=w369:T6, "Result.error"=w367:errorcluster)
        n133 = case shown="No Error" w367 {
          tunnel: w370 -> [w377 _]
          tunnel: w369 -> [w376 _]
          tunnel: w368 -> [w375 _]
          frame No Error {
            n134 = case shown="True" w375 {
              tunnel: w376 -> [_ w381]
              tunnel: w377 -> [_ w380]
              frame False {
              }
              frame True {
                n135 = property class="VI"(reference=w380, "FP.State"=w381) -> (reference out=w378:refnum<vi>, error out=w379:errorcluster)  [unwired: 1 in]
                n136 = call "Safely Close Reference - Half Height_nevstop.vim"("error in (no error)"=w379, "Reference"=w378) -> ()  [unwired: 9 in, 1 out]
              }
            }
          }
          frame Error {
          }
        }
      }
      frame "UI: Set Titlebar State" {
        n137 = Unbundle By Name(w384) -> ("Core.Current VI Reference"=w383:refnum<vi>, "Options.Titlebar(T)"=w382:bool)
        n138 = property class="VI"(reference=w383, "Front Panel.TitleBarVis"=w382) -> ()  [unwired: 1 in, 2 out]
      }
      frame "---------- Macro ----------" {
        # "Do not put any code in this frame.\n(It is a separator no-op. You can make a copy of this frame to create a new Macro frame)"
        n139 = call <vilib>:"Add State(s) to Queue__JKI_lib_State_Machine.vi"("State(s) in (\"\")"=w392) -> ("States Out"=w391:string)  [unwired: 14 in]
      }
      frame "Macro: Initialize" {
        # "Initialization Macro\n(This is called once, when the VI starts)"
        n140 = call <vilib>:"Add State(s) to Queue__JKI_lib_State_Machine.vi"("State(s) in Front (\"\")"="Data: Initialize\nInitialize Core Data\nEvents: Register\nUI: Initialize\n//UI: Front Panel State >> Open", "State(s) in (\"\")"=w398) -> ("States Out"=w397:string)  [unwired: 13 in]
      }
      frame "Macro: Exit" {
        # "Exit Macro\n(This is called once, when the VI exits)"
        n141 = Unbundle By Name(w406) -> ("Core.Close Panel on Exit?"=w405:bool)
        n142 = Select(t="UI: Front Panel State >> Close", s=w405, f="") -> (s? t:f=w402:string)
        n143 = call <vilib>:"Add State(s) to Queue__JKI_lib_State_Machine.vi"("State(s) in (\"\")"=w402, "State(s) at Back (\"\")"="UI: Restore Caller Panel State\nData: Set LastLoginUser\nData: Cleanup\nEvents: Unregister\nExit") -> ("States Out"=w400:string)  [unwired: 13 in]
        n144 = call <vilib>:"Add State(s) to Queue__JKI_lib_State_Machine.vi"("State(s) in Front (\"\")"=w400, "State(s) in (\"\")"=w409) -> ("States Out"=w408:string)  [unwired: 13 in]
      }
      frame "---------- Action ----------" {
        # "Template Separator\n(You can make a copy of, or modify, this frame)"
        n145 = call <vilib>:"Add State(s) to Queue__JKI_lib_State_Machine.vi"("State(s) in (\"\")"=w414) -> ("States Out"=w413:string)  [unwired: 14 in]
      }
      frame "Action: Login" {
        n146 = Unbundle By Name(w425) -> ("Options.RetryAllowed(T)"=w427:bool, "UserName"=w424:string, "Password"=w423:string)
        n147 = Bundle By Name(cluster=T3 {"UserName"="", "Password"="", "Role"=enum."Admin"} ("Userinfo"), "UserName"=w424, "Password"=w423) -> (w417:T3)
        n148 = Not(x=w427) -> (.not. x?=w428:bool)
        n149 = call-dynamic "Validate.vi"("PwdMgr in"=w418, "Cluster"=w417) -> ("error out"=w429:errorcluster, "Valid?"=w415:bool, "Userinfo out"=w416:T3)  [unwired: 7 in]
        n150 = case shown="False" w415 {
          tunnel: w429 -> [_ w438]
          tunnel: [w435 w438] -> w420
          frame False {
            w436 = "UserName or Password is Wrong." ("message")
            n151 = One Button Dialog(message=w436) -> ()  [unwired: 1 in, 1 out]
            n152 = Bundle(TRUE, "code"=-1, "message"=w436) -> (w435:cluster{bool, "code":i32, "message":string})  [unwired: 1 in]
          }
          frame True {
          }
        }
        n153 = Or(x=w415, y=w428) -> (x .or. y?=w419:bool)
        n154 = Bundle By Name(cluster=w425, "Result.LoginSuccess"=w415, "Result.error"=w420, "Result.User Info"=w416) -> (w421:T8)
        n155 = call <userlib>:"JKI Insert State by Bool_nevstop.vi"("TRUE(Empty)"="Macro: Exit", "Bool"=w419, "Remaining States"=w433) -> ("States Out"=w432:string)  [unwired: 8 in]
      }
      frame "Action: Anonymous Login" {
        w440 = TRUE ("Bool")
        # "#GitHub 12\n支持匿名登录"
        n156 = Bundle By Name(cluster=w443, "Result.LoginSuccess"=w440, "Result.User Info"=T3 {"UserName"="anonymous", "Password"="", "Role"=enum."Anonymous"}) -> (w441:T8)
        n157 = call <userlib>:"JKI Insert State by Bool_nevstop.vi"("TRUE(Empty)"="Macro: Exit", "Bool"=w440, "Remaining States"=w447) -> ("States Out"=w446:string)  [unwired: 8 in]
      }
      frame "Action: Action: UserManage" {
        n158 = Unbundle By Name(w456) -> ("UserName"=w455:string, "Password"=w454:string)
        n159 = Bundle By Name(cluster=T3 {"UserName"="", "Password"="", "Role"=enum."Admin"} ("Userinfo"), "UserName"=w455, "Password"=w454) -> (w451:T3)
        n160 = call-dynamic "Validate.vi"("PwdMgr in"=w448, "Cluster"=w451) -> ("error out"=w453:errorcluster, "Valid?"=w449:bool, "Userinfo out"=w450:T3)  [unwired: 7 in]
        n161 = case shown="True" w449 {
          tunnel: w453 -> [_ w468]
          tunnel: [w462 w467] -> w452
          tunnel: w450 -> [_ w465]
          tunnel: w448 -> [_ w464]
          frame False {
            n162 = Bundle(TRUE, "code"=-1, "String to Prepend to source (\"\")"="UserName or Password is Wrong." ("String to Prepend to source (\"\")")) -> (w462:T11)  [unwired: 1 in]
          }
          frame True {
            n163 = Unbundle By Name(w465) -> ("Role"=w466:T4)
            n164 = case shown="\"INVALID\"" w466 {
              tunnel: w468 -> [_ w475 w478]
              tunnel: [w470 w474 w477] -> w467
              tunnel: w465 -> [_ w473 _]
              tunnel: w464 -> [_ w472 w476]
              frame "INVALID" {
                n165 = call <userlib>:"Error From Error Code_nevstop.vi"("error message (\"\")"="没有权限" ("String to Prepend to source (\"\")"), "error code (0)"=-1 ("code")) -> ("error out"=w470:errorcluster)  [unwired: 7 in]
              }
              frame Default {
                n166 = call "ChangePassword-Window.vi"("PwdMgr"=w472, "error in (no error)"=w475, "User Info"=w473) -> ("error out"=w474:errorcluster)  [unwired: 8 in]
              }
              frame "Admin" {
                n167 = call "UserMgr-Window.vi"("PwdMgr"=w476, "error in"=w478) -> ("error out"=w477:errorcluster)  [unwired: 9 in]
              }
            }
          }
        }
      }
    }
  }
  n168 = Unbundle By Name(w7) -> ("Result.LoginSuccess"=→"Valid User":bool, "Result.error"=w5:errorcluster, "Result.User Info"=→"User Info":T3)
  n169 = Merge Errors(w8, w5) -> (→"Error out":errorcluster)
